vi "Line Follower 2.vi"() -> ()   [LabVIEW 2015]
uses:
  <vilib>/myRIO/Instrument Drivers/Onboard IO/AI/typedefs/AI Reference.ctl
  <vilib>/myRIO/Common/Instrument Driver Framework/Utilities/typedefs/myRIO Generic Hardware Reference.ctl
  <vilib>/myRIO/Common/Instrument Driver Framework/Utilities/typedefs/Hardware Version Enum.ctl
  <vilib>/myRIO/Common/Instrument Driver Framework/Utilities/typedefs/myRIO v1.0 Reference.ctl
  <vilib>/myRIO/Common/Instrument Driver Framework/Utilities/typedefs/Generic FPGA Reference.ctl
  <vilib>/myRIO/Common/Instrument Driver Framework/myRIO v1.0/AI/typedefs/AI Channels List.ctl
  <vilib>/myRIO/Common/Instrument Driver Framework/myRIO v1.0/AI/typedefs/AI Channels Enum.ctl
  <vilib>/myRIO/Common/Instrument Driver Framework/Utilities/typedefs/Analog Scaling Constants List.ctl
  <vilib>/myRIO/Common/Instrument Driver Framework/Utilities/typedefs/Analog Scaling Constants.ctl
  <vilib>/userdefined/High Color/nirio_resource_hc.ctl
  <vilib>/myRIO/Common/Instrument Driver Framework/Utilities/vis/Is FPGA Ref Available.vi
  <vilib>/myRIO/Common/Instrument Driver Framework/myRIO v1.0/AI/vis/myRIO v1.1 Open AI.vi
  <vilib>/myRIO/Instrument Drivers/Onboard IO/AI/vis/Read.vi
  <vilib>/myRIO/Common/Instrument Driver Framework/Utilities/vis/Validate Channels.vi
  <vilib>/myRIO/Common/Instrument Driver Framework/myRIO v1.0/AI/vis/myRIO v1.0 Reserve AI.vi
  <vilib>/myRIO/Common/Instrument Driver Framework/myRIO v1.0/AI/vis/myRIO v1.0 Build MUX Configuration AI.vi
  <vilib>/myRIO/Common/Instrument Driver Framework/myRIO v1.0/Resource Manager/vis/myRIO v1.0 Reserve Channel List.vi
  <vilib>/myRIO/Common/Instrument Driver Framework/myRIO v1.0/Resource Manager/vis/myRIO v1.0 Reserve Channel.vi
  <vilib>/myRIO/Common/Instrument Driver Framework/myRIO v1.0/Resource Manager/vis/myRIO v1.0 Unreserve Channel.vi
  <vilib>/myRIO/Common/Instrument Driver Framework/myRIO v1.0/Resource Manager/vis/myRIO v1.0 Build Mutex Name.vi
  <vilib>/Utility/VariantDataType/GetNumericInfo.vi
  <vilib>/Utility/error.llb/Error Cluster From Error Code.vi
  <vilib>/myRIO/Common/Instrument Driver Framework/myRIO v1.0/myRIO v1.1 Open.vi
  <vilib>/myRIO/Common/Instrument Driver Framework/myRIO v1.0/AI/vis/myRIO v1.0 Get Scaling Constants AI.vi
  <vilib>/myRIO/Common/Instrument Driver Framework/Utilities/vis/IO Manager.vi
  <vilib>/myRIO/Common/Instrument Driver Framework/Utilities/vis/Configuration Manager.vi
  <vilib>/myRIO/Common/Instrument Driver Framework/myRIO v1.0/myRIO v1.0 Close.vi
  <vilib>/myRIO/Common/Instrument Driver Framework/myRIO v1.0/AI/vis/myRIO v1.0 Read AI.vi
  <vilib>/myRIO/Express VI/Onboard IO/AI/AI Express VI.xnode
  <vilib>/myRIO/Instrument Drivers/Onboard IO/AI/vis/myRIO AI Open.xnode
  <vilib>/myRIO/Instrument Drivers/Onboard IO/AI/AI.lvlib
panel:
  in  "U":dbl
  in  "last error":dbl
  in  "D":dbl
  in  "integral":dbl
  in  "error":dbl
  in  "speed":dbl
  in  "P":dbl
  in  "I":dbl
  out "front left":i16
  out "front right":i16
  out "back left":i16
  out "back right":i16
  out "left read":dbl
  out "right read":dbl
  in  "stop":bool
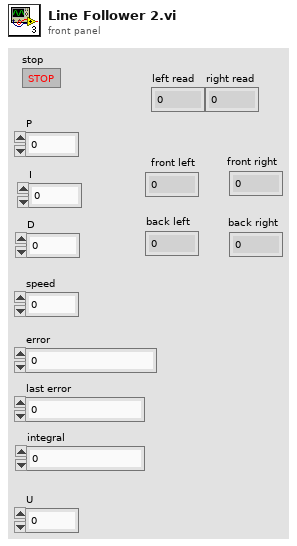
[diagram p1: front panel]
types:
  T1 = typedef "AI.lvlib/AI Reference.ctl" = cluster{"myRIO Reference":T2, "AI Channels List":T6, "AI Scaling Constants List":T8}
  T2 = typedef "myRIO Generic Hardware Reference.ctl" = cluster{"myRIO Model":T3, "myRIO Hardware Reference":T4}
  T3 = typedef "Hardware Version Enum.ctl" = enum16{"Unknown", "myRIO-1900", "myRIO-1950", "roboRIO"}
  T4 = typedef "myRIO v1.0 Reference.ctl" = cluster{"Generic FPGA Reference":T5, "Allow multiple opens":bool}
  T5 = typedef "Generic FPGA Reference.ctl" = refnum<k20>
  T6 = typedef "AI Channels List.ctl" = T7[]
  T7 = typedef "AI Channels Enum.ctl" = enum16{"Not Connected", "AudioIn/Left", "AudioIn/Right", "C/AI0", "C/AI1", "A/AI0", "A/AI1", "A/AI2", "A/AI3", "B/AI0", "B/AI1", "B/AI2", "B/AI3", "AI/AI0", "AI/AI1", "AI/AI2", "AI/AI3"}
  T8 = typedef "Analog Scaling Constants List.ctl" = T9[]
  T9 = typedef "Analog Scaling Constants.ctl" = cluster{"LSB Weight (Volts)":dbl, "Offset (Volts)":dbl, "Signed?":bool}
  T10 = typedef "nirio_resource_hc.ctl" = tag
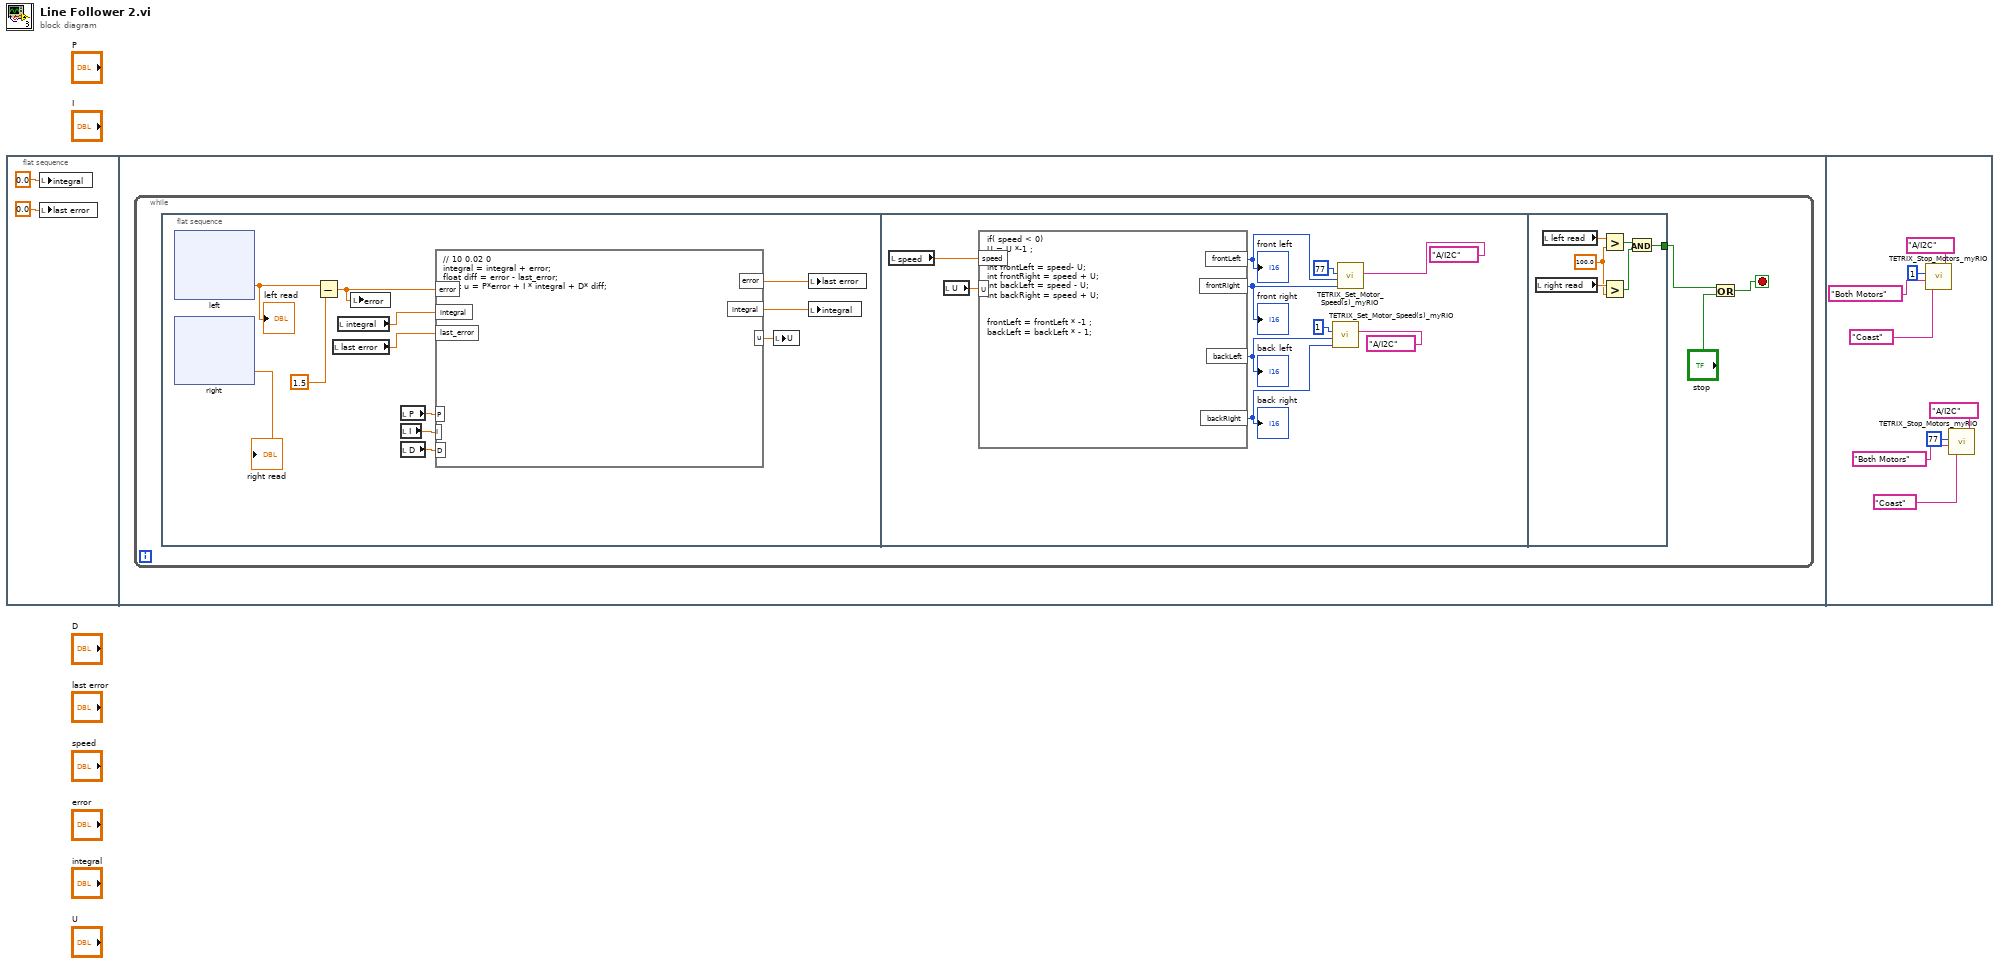
[diagram p0: block diagram]
diagram:
  n1 = flat-sequence {
    frame #0 {
      n2 = local write "integral"(0.0 ("integral")) -> ()
      n3 = local write "last error"(0.0 ("last error")) -> ()
    }
    frame #1 {
      n4 = while {
        stop <- w3 stop-if-true
        n5 = flat-sequence {
          tunnel: [w102] -> w5
          frame #0 {
            n6 = xnode "left"() -> ("A/AI0 (Pin 3)"=w17:dbl)  [unwired: 1 in, 1 out]
            "left read" <- w17
            n7 = xnode "right"() -> ("A/AI1 (Pin 5)"=→"right read":dbl)  [unwired: 1 in, 1 out]
            n8 = Subtract(x=w17, y=1.5) -> (x-y=w12:dbl)
            n9 = local read "last error"() -> (w10:dbl)
            n10 = local read "integral"() -> (w11:dbl)
            n11 = local write "error"(w12) -> ()
            n12 = local read "P"() -> (w9:dbl)
            n13 = local read "I"() -> (w8:dbl)
            n14 = local read "D"() -> (w7:dbl)
            n15 = formula code="// 10 0.02 0\nintegral = integral + error;\nfloat diff = error - last_error;\nfloat u = P*error + I * integral + D* diff;"("error"=w12, "integral"=w11, "last_error"=w10, "P"=w9, "I"=w8, "D"=w7) -> ("error"=w15:dbl, "integral"=w14:dbl, "u"=w13:dbl)
            n16 = local write "U"(w13) -> ()
            n17 = local write "last error"(w15) -> ()
            n18 = local write "integral"(w14) -> ()
          }
          frame #1 {
            n19 = local read "speed"() -> (w93:dbl)
            n20 = local read "U"() -> (w92:dbl)
            n21 = formula code="if( speed < 0)\nU = U *-1 ;\n\nint frontLeft = speed- U;\nint frontRight = speed + U;\nint backLeft = speed - U;\nint backRight = speed + U;\n\n\nfrontLeft = frontLeft * -1 ;\nbackLeft = backLeft * - 1;"("speed"=w93, "U"=w92) -> ("frontLeft"=w97:i32, "frontRight"=w96:i32, "backLeft"=w95:i32, "backRight"=w94:i32)
            "front left" <- w97
            "front right" <- w96
            "back left" <- w95
            "back right" <- w94
            n22 = call <vilib>:"TETRIX_Set_Motor_Speed(s)_myRIO.vi"("myRIO MXP Port A/B"=tag "A/I2C", "Motor 2 Speed (Degrees per second). Sign (+/-)  sets direction."=w94, "Motor 1 Speed (Degrees per second). Sign (+/-)  sets direction."=w95, "Controller ID#  (I2C Address)"=u8 1) -> ()  [unwired: 3 in, 1 out]
            n23 = call <vilib>:"TETRIX_Set_Motor_Speed(s)_myRIO.vi"("myRIO MXP Port A/B"=tag "A/I2C", "Motor 2 Speed (Degrees per second). Sign (+/-)  sets direction."=w96, "Motor 1 Speed (Degrees per second). Sign (+/-)  sets direction."=w97, "Controller ID#  (I2C Address)"=u8 77) -> ()  [unwired: 3 in, 1 out]
          }
          frame #2 {
            w105 = 100.0 ("y")
            n24 = local read "right read"() -> (w106:dbl)
            n25 = local read "left read"() -> (w107:dbl)
            n26 = Greater?(x=w107, y=w105) -> (0:w104:bool)
            n27 = Greater?(x=w106, y=w105) -> (0:w103:bool)
            n28 = And(x=w104, y=w103) -> (x .and. y?=w102:bool)
          }
        }
        n29 = Or(x=w5, y="stop") -> (x .or. y?=w3:bool)
      }
    }
    frame #2 {
      n30 = call <vilib>:"TETRIX_Stop_Motors_myRIO.vi"("myRIO MXP Port A/B"=tag "A/I2C", "Stop Mode"="Coast", "Select Channel"="Both Motors", "Controller ID#  (I2C Address)"=u8 1) -> ()  [unwired: 3 in, 1 out]
      n31 = call <vilib>:"TETRIX_Stop_Motors_myRIO.vi"("myRIO MXP Port A/B"=tag "A/I2C", "Stop Mode"="Coast", "Select Channel"="Both Motors", "Controller ID#  (I2C Address)"=u8 77) -> ()  [unwired: 3 in, 1 out]
    }
  }
